vi "Monitored Actor Switcher.vi"() -> ()   [LabVIEW 2017]
doc: "Provides an easy way to switch actors between monitored actors and reular actors\n\nCopyright: Hill\nAuthored by: Derek Trepanier"
panel:
  in  "Non Actors":i32[](listbox)
  in  "All Actors to Non":bool
  in  "Actor to Non":bool
  in  "All Non to Actors":bool
  in  "Non to Actor":bool
  in  "Actors":i32[](listbox) caption="MGI-Monitored Actor Core.lvlib:Actor Monitor.lvclass"
  in  "All Mon to Actors":bool
  in  "Mon to Actor":bool
  in  "All Actors to Mon":bool
  in  "Actor To Mon":bool
  in  "Monitored Actors":i32[](listbox) caption="Example Actor.lvlib:Example Actor.lvclass"
  in  "Include Items in Dependancies?":bool
  in  "Cancel":bool
  in  "Save":bool
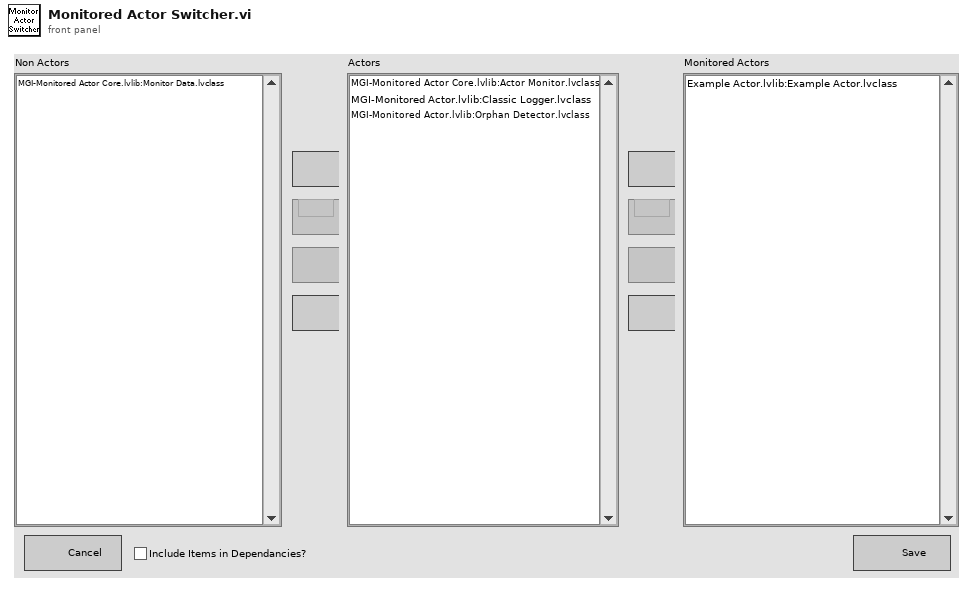
[diagram p1: front panel]
types:
  T1 = enum8{"Enabled", "Disabled", "Disabled and Grayed Out"}
  T2 = typedef "LVPoint32TypeDef.ctl" = cluster{"Horizontal":i32, "Vertical":i32}
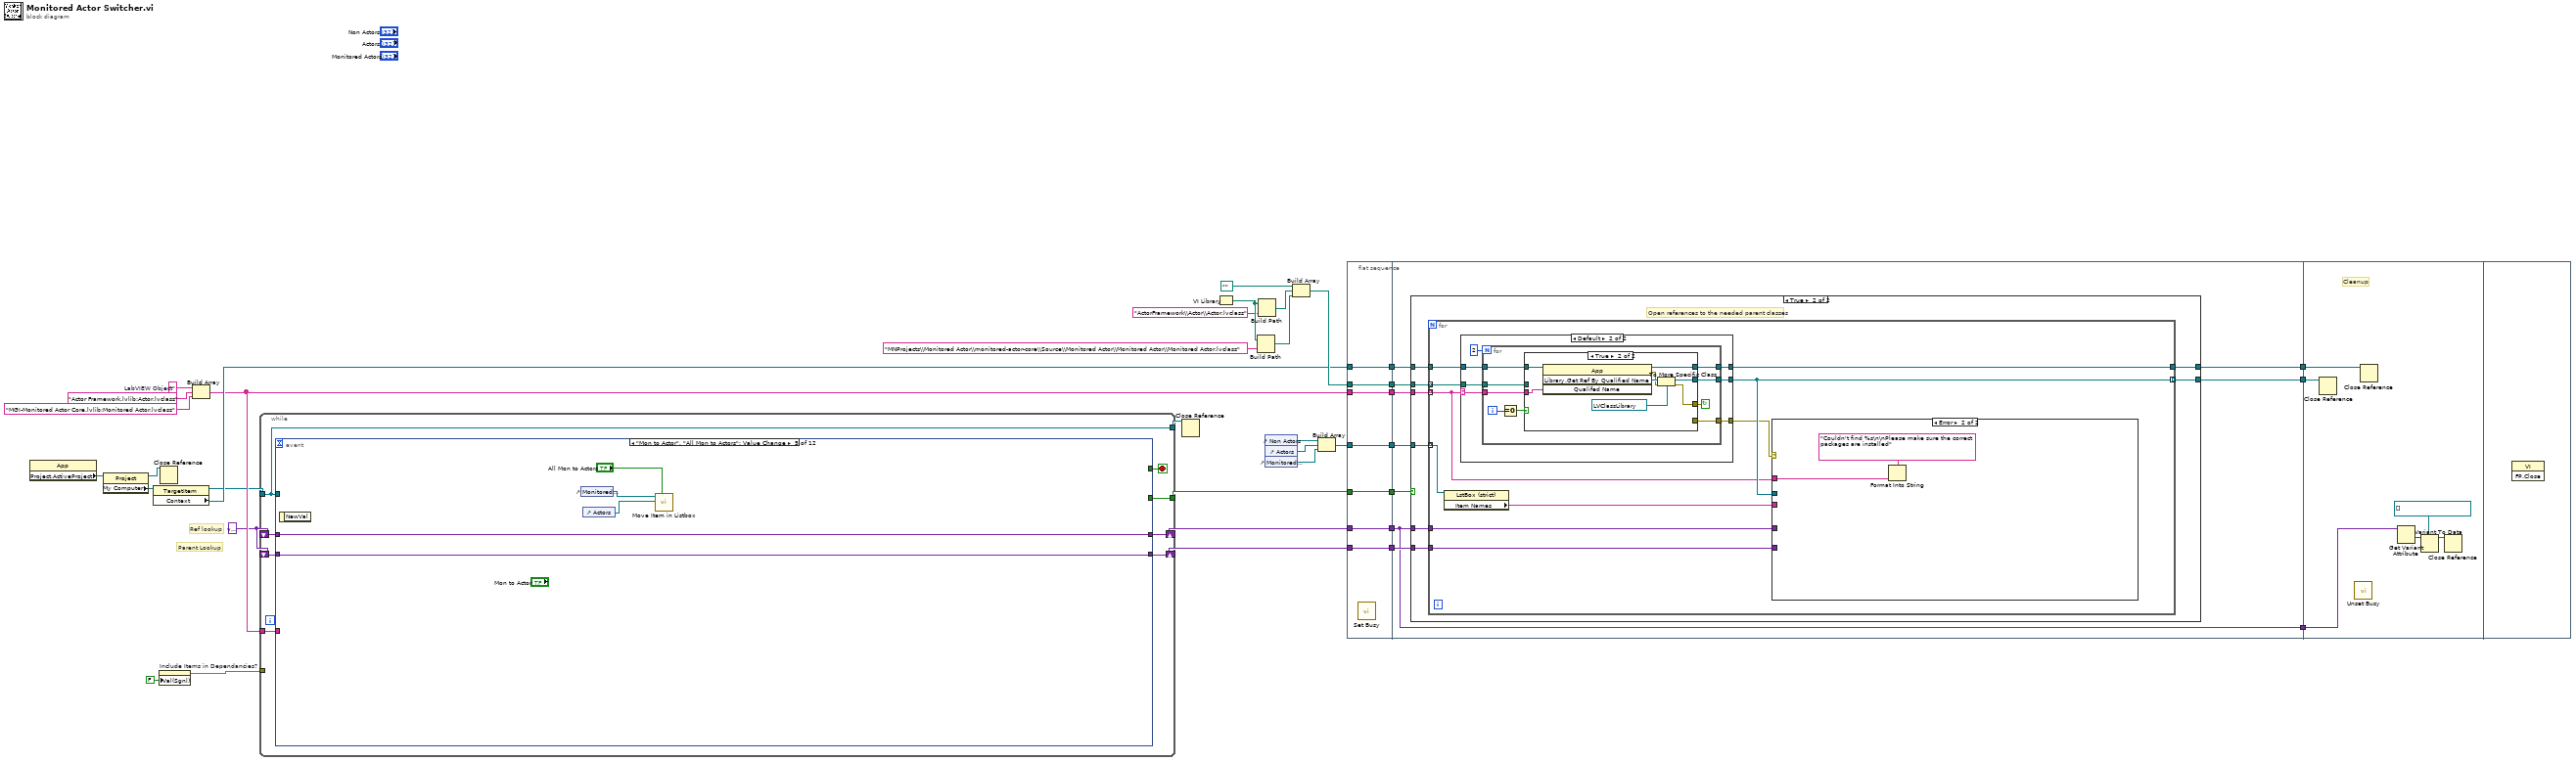
[diagram p0: block diagram]
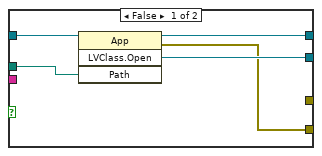
[diagram p4: hidden frame]
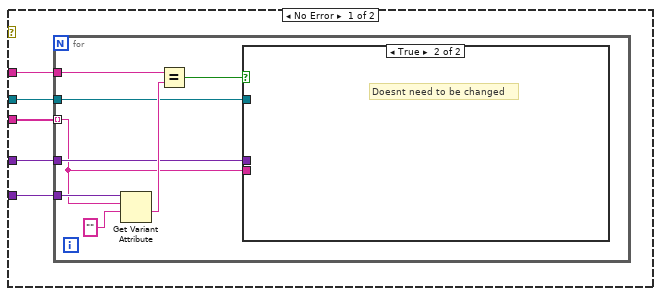
[diagram p5: hidden frame]
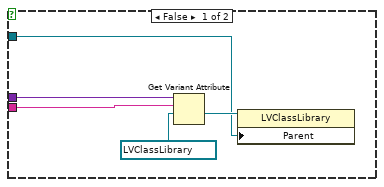
[diagram p6: hidden frame]
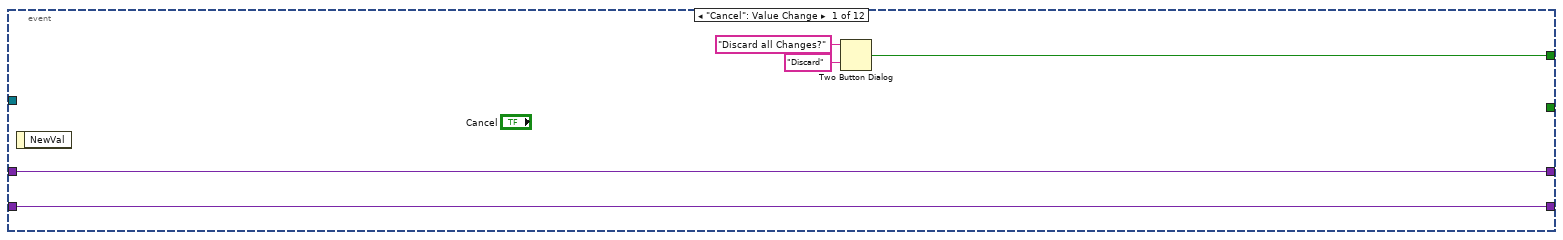
[diagram p7: hidden frame]
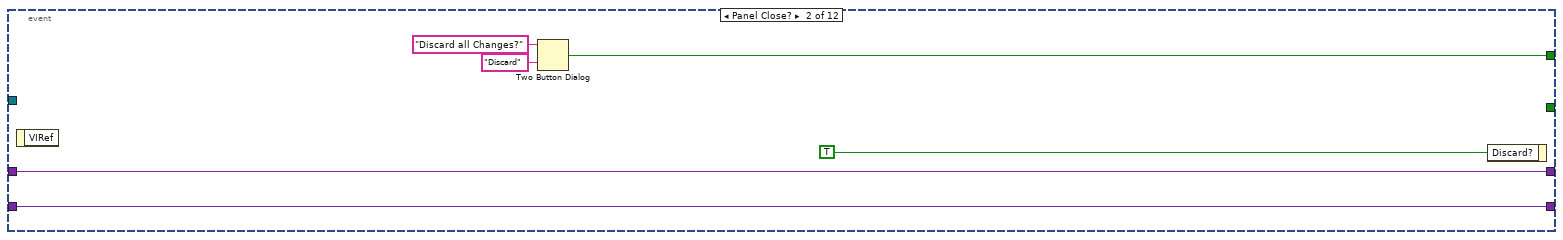
[diagram p8: hidden frame]
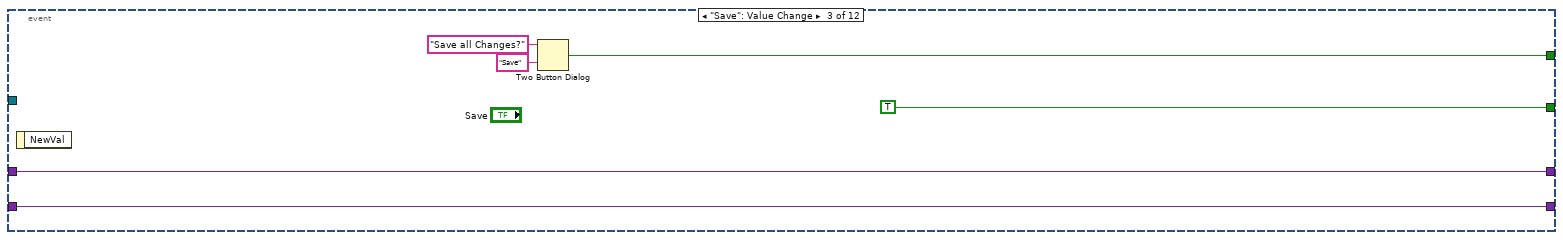
[diagram p9: hidden frame]
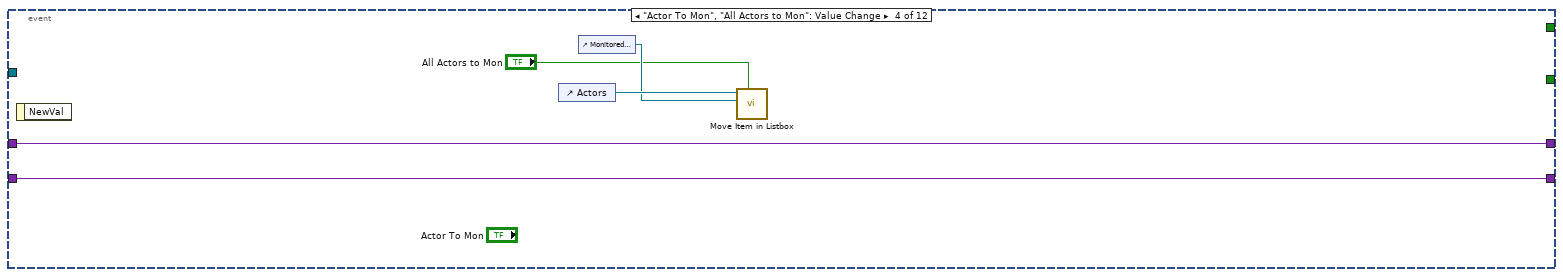
[diagram p10: hidden frame]
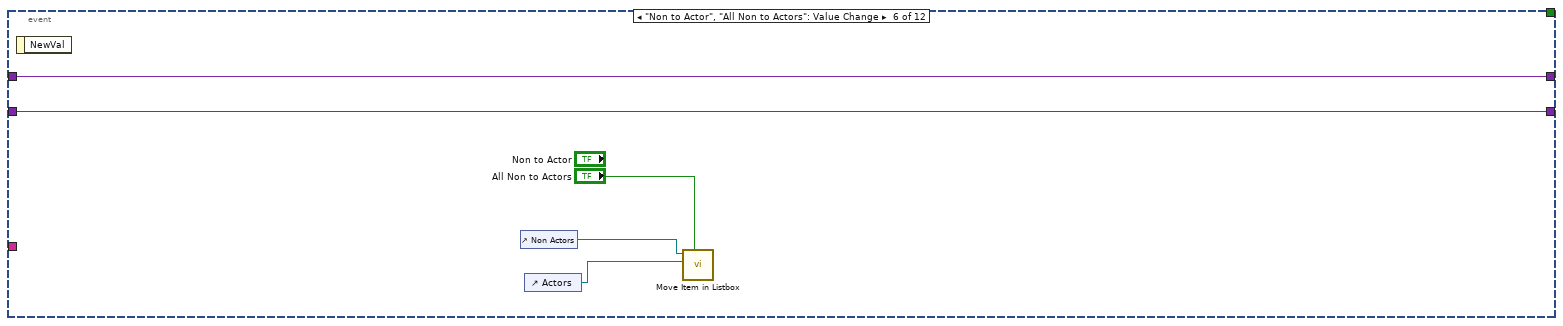
[diagram p11: hidden frame]
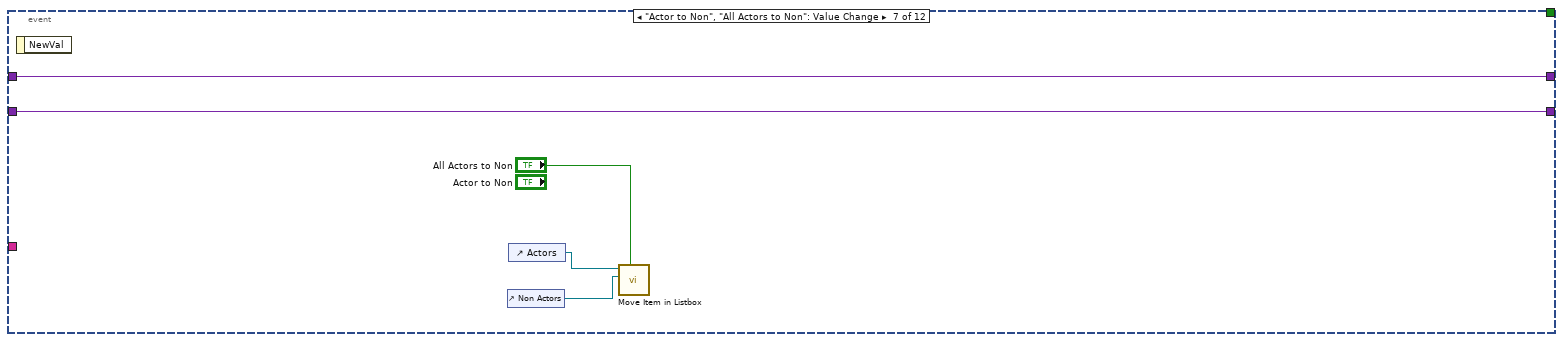
[diagram p12: hidden frame]
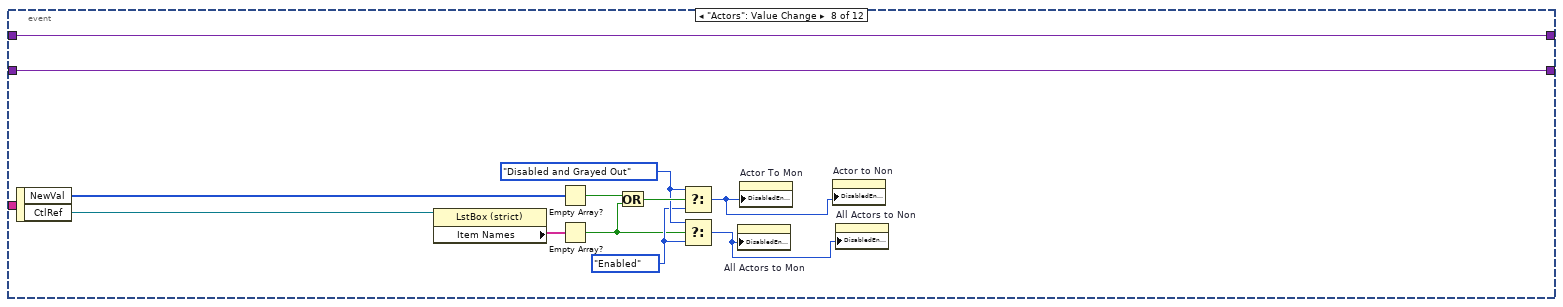
[diagram p13: hidden frame]
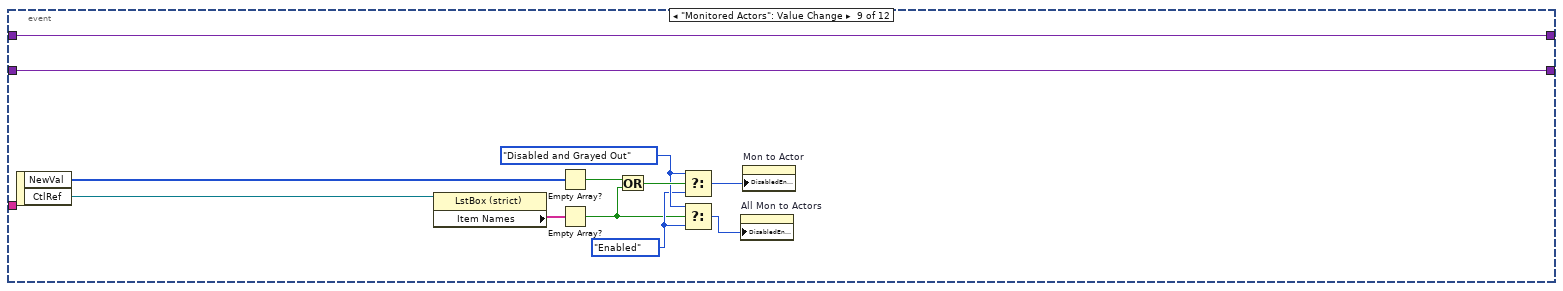
[diagram p14: hidden frame]
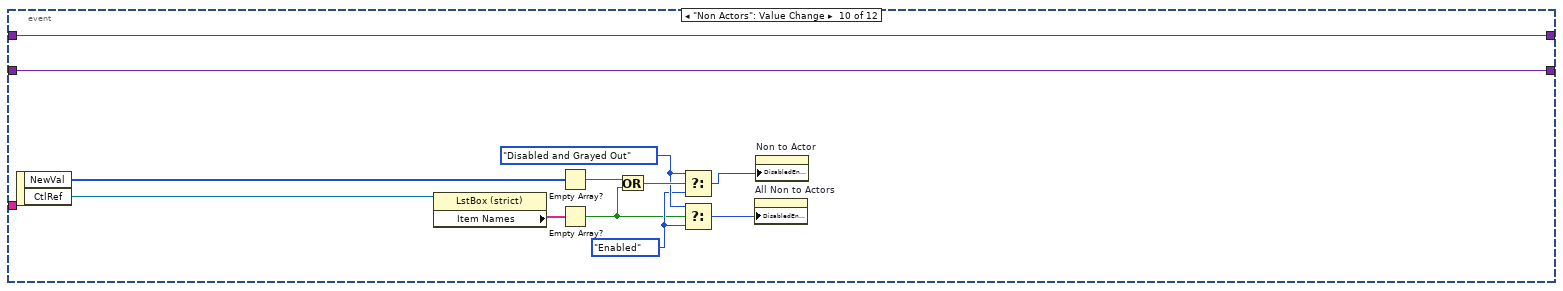
[diagram p15: hidden frame]
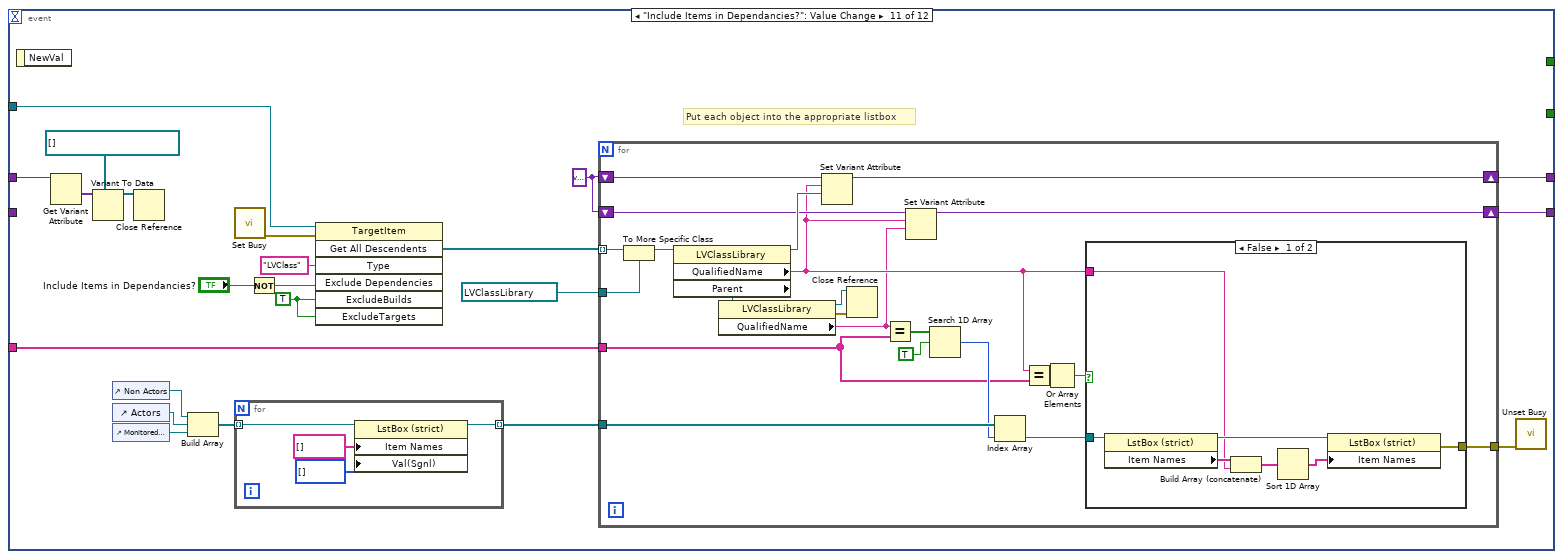
[diagram p16: hidden frame]
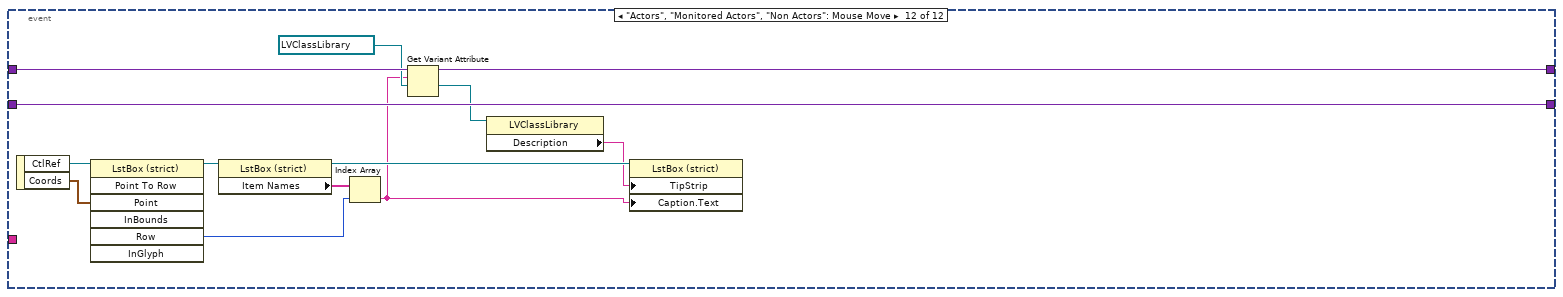
[diagram p18: hidden frame]
diagram:
  w1 = variant ("Variant")
  w11 = ""  # LabVIEW Object
  # "Parent Lookup"
  # "Ref lookup"
  n1 = property class="App"() -> ("Project.ActiveProject"=w37:refnum<vi>)  [unwired: 2 in, 2 out]
  n2 = property class="Project"(reference=w37) -> (reference out=w35:refnum<vi>, "My Computer"=w36:refnum<vi>)  [unwired: 1 in, 1 out]
  n3 = property class="TargetItem"(reference=w36) -> (reference out=w5:refnum<vi>, "Context"=w30:refnum<vi>)  [unwired: 1 in, 1 out]
  n4 = property on="Include Items in Dependancies?" class="Bool (strict)"("Val(Sgnl)"=FALSE ("Value (Signaling)")) -> (error out=w3:errorcluster)  [unwired: 2 in, 1 out]
  n5 = Close Reference(reference=w35) -> ()  [unwired: 1 in, 1 out]
  n6 = Build Array(w11, "Actor Framework.lvlib:Actor.lvclass" ("Qualified Name"), "MGI-Monitored Actor Core.lvlib:Monitored Actor.lvclass" ("Qualified Name")) -> (w8:string[])
  n7 = while {
    tunnel: [w44] -> w22
    tunnel: w8 -> [w43]
    tunnel: w5 -> [w40]
    tunnel: w3 -> [_]
    tunnel: [w40] -> w2
    shift-right: [w42] -> w7
    shift-left: w1 -> [w38]
    shift-right: [w41] -> w6
    shift-left: w1 -> [w39]
    stop <- w45 stop-if-true
    n8 = event shown="[4] \"Mon to Actor\", \"All Mon to Actors\": Value Change" {
      selector: _ -> [_ _ _ _ _ _ _ _ _ _ _ _]
      dyn-events: _ -> [_ _ _ _ _ _ _ _ _ _ _ _]
      timeout: _ -> [_ _ _ _ _ _ _ _ _ _ _ _]
      tunnel: [w50 w56 w62 _ _ _ _ _ _ _ _ _] -> w45
      tunnel: [_ _ TRUE _ _ _ _ _ _ _ _ _] -> w44
      tunnel: w43 -> [_ _ _ _ _ _ _ _ _ _ w130 _]
      tunnel: [w47 w52 w58 w64 w69 w74 w79 w84 w96 w108 w128 w179] -> w42
      tunnel: [w46 w51 w57 w63 w68 w73 w78 w83 w95 w107 w127 w186] -> w41
      tunnel: w40 -> [_ _ _ _ _ _ _ _ _ _ w125 _]
      tunnel: w39 -> [w46 w51 w57 w63 w68 w73 w78 w83 w95 w107 _ w186]
      tunnel: w38 -> [w47 w52 w58 w64 w69 w74 w79 w84 w96 w108 w119 w180]
      event "Cancel": Value Change {
        n9 = event-data() -> ()  [unwired: 1 in, 1 out]
        n10 = Two Button Dialog(message="Discard all Changes?", 2:"Discard" ("T button name (\"OK\")")) -> (T button?=w50:bool)  [unwired: 1 in]
      }
      event Panel Close? {
        n11 = event-data() -> ()  [unwired: 1 in, 1 out]
        n12 = Two Button Dialog(message="Discard all Changes?", 2:"Discard" ("T button name (\"OK\")")) -> (T button?=w56:bool)  [unwired: 1 in]
        n13 = event-data("Discard?"=TRUE) -> ()  [unwired: 1 in, 1 out]
      }
      event "Save": Value Change {
        n14 = event-data() -> ()  [unwired: 1 in, 1 out]
        n15 = Two Button Dialog(message="Save all Changes?", 2:"Save" ("T button name (\"OK\")")) -> (T button?=w62:bool)  [unwired: 1 in]
      }
      event "Actor To Mon", "All Actors to Mon": Value Change {
        n16 = event-data() -> ()  [unwired: 1 in, 1 out]
        n17 = control-ref of="Actors"() -> (w67:refnum<vi>)
        n18 = control-ref of="Monitored Actors"() -> (w66:refnum<vi>)
        n19 = call "Move Item in Listbox.vi"("Move All Items? (f)"="All Actors to Mon", "Destination Lisbox"=w66, "Source Listbox"=w67) -> ()  [unwired: 9 in]
      }
      event "Mon to Actor", "All Mon to Actors": Value Change {
        n20 = event-data() -> ()  [unwired: 1 in, 1 out]
        n21 = control-ref of="Monitored Actors"() -> (w70:refnum<vi>)
        n22 = control-ref of="Actors"() -> (w71:refnum<vi>)
        n23 = call "Move Item in Listbox.vi"("Move All Items? (f)"="All Mon to Actors", "Destination Lisbox"=w71, "Source Listbox"=w70) -> ()  [unwired: 9 in]
      }
      event "Non to Actor", "All Non to Actors": Value Change {
        n24 = event-data() -> ()  [unwired: 1 in, 1 out]
        n25 = control-ref of="Non Actors"() -> (w77:refnum<vi>)
        n26 = control-ref of="Actors"() -> (w76:refnum<vi>)
        n27 = call "Move Item in Listbox.vi"("Move All Items? (f)"="All Non to Actors", "Destination Lisbox"=w76, "Source Listbox"=w77) -> ()  [unwired: 9 in]
      }
      event "Actor to Non", "All Actors to Non": Value Change {
        n28 = event-data() -> ()  [unwired: 1 in, 1 out]
        n29 = control-ref of="Non Actors"() -> (w80:refnum<vi>)
        n30 = control-ref of="Actors"() -> (w81:refnum<vi>)
        n31 = call "Move Item in Listbox.vi"("Move All Items? (f)"="All Actors to Non", "Destination Lisbox"=w80, "Source Listbox"=w81) -> ()  [unwired: 9 in]
      }
      event "Actors": Value Change {
        w88 = T1."Enabled" ("Disabled")
        w89 = T1."Disabled and Grayed Out" ("Disabled")
        n32 = event-data() -> ("NewVal"=w94:i32[], "CtlRef"=w93:refnum<vi>)  [unwired: 1 in]
        n33 = property class="LstBox (strict)"(reference=w93) -> ("Item Names"=w92:string[])  [unwired: 1 in, 2 out]
        n34 = Empty Array?(array=w94) -> (empty?=w91:bool)
        n35 = Empty Array?(array=w92) -> (empty?=w87:bool)
        n36 = Or(x=w91, y=w87) -> (x .or. y?=w90:bool)
        n37 = Select(t=w89, s=w90, f=w88) -> (s? t:f=w85:T1)
        n38 = Select(t=w89, s=w87, f=w88) -> (s? t:f=w86:T1)
        n39 = property on="All Actors to Mon" class="Bool"("DisabledEnum"=w86) -> ()  [unwired: 2 in, 2 out]
        n40 = property on="Actor To Mon" class="Bool"("DisabledEnum"=w85) -> ()  [unwired: 2 in, 2 out]
        n41 = property on="Actor to Non" class="Bool"("DisabledEnum"=w85) -> ()  [unwired: 2 in, 2 out]
        n42 = property on="All Actors to Non" class="Bool"("DisabledEnum"=w86) -> ()  [unwired: 2 in, 2 out]
      }
      event "Monitored Actors": Value Change {
        w100 = T1."Enabled" ("Disabled")
        w101 = T1."Disabled and Grayed Out" ("Disabled")
        n43 = event-data() -> ("NewVal"=w106:i32[], "CtlRef"=w105:refnum<vi>)  [unwired: 1 in]
        n44 = property class="LstBox (strict)"(reference=w105) -> ("Item Names"=w104:string[])  [unwired: 1 in, 2 out]
        n45 = Empty Array?(array=w106) -> (empty?=w103:bool)
        n46 = Empty Array?(array=w104) -> (empty?=w99:bool)
        n47 = Or(x=w103, y=w99) -> (x .or. y?=w102:bool)
        n48 = Select(t=w101, s=w102, f=w100) -> (s? t:f=w98:T1)
        n49 = Select(t=w101, s=w99, f=w100) -> (s? t:f=w97:T1)
        n50 = property on="All Mon to Actors" class="Bool"("DisabledEnum"=w97) -> ()  [unwired: 2 in, 2 out]
        n51 = property on="Mon to Actor" class="Bool"("DisabledEnum"=w98) -> ()  [unwired: 2 in, 2 out]
      }
      event "Non Actors": Value Change {
        w112 = T1."Enabled" ("Disabled")
        w113 = T1."Disabled and Grayed Out" ("Disabled")
        n52 = event-data() -> ("NewVal"=w118:i32[], "CtlRef"=w117:refnum<vi>)  [unwired: 1 in]
        n53 = property class="LstBox (strict)"(reference=w117) -> ("Item Names"=w116:string[])  [unwired: 1 in, 2 out]
        n54 = Empty Array?(array=w118) -> (empty?=w115:bool)
        n55 = Empty Array?(array=w116) -> (empty?=w111:bool)
        n56 = Or(x=w115, y=w111) -> (x .or. y?=w114:bool)
        n57 = Select(t=w113, s=w114, f=w112) -> (s? t:f=w109:T1)
        n58 = Select(t=w113, s=w111, f=w112) -> (s? t:f=w110:T1)
        n59 = property on="All Non to Actors" class="Bool"("DisabledEnum"=w110) -> ()  [unwired: 2 in, 2 out]
        n60 = property on="Non to Actor" class="Bool"("DisabledEnum"=w109) -> ()  [unwired: 2 in, 2 out]
      }
      event "Include Items in Dependancies?": Value Change {
        w140 = variant ("Variant")
        w139 = TRUE ("ExcludeDependencies")
        # "Put each object into the appropriate listbox"
        n61 = event-data() -> ()  [unwired: 1 in, 1 out]
        n62 = Get Variant Attribute(Variant=w119) -> (values=w121:variant[])  [unwired: 3 in, 3 out]
        n63 = Variant To Data(type=refnum<vi>[] [] ("Children In Memory[]"), Variant=w121) -> (data=w120:refnum<vi>[])  [unwired: 1 in, 1 out]
        n64 = control-ref of="Non Actors"() -> (w133:refnum<vi>)
        n65 = control-ref of="Actors"() -> (w131:refnum<vi>)
        n66 = control-ref of="Monitored Actors"() -> (w132:refnum<vi>)
        n67 = Close Reference(reference=w120) -> ()  [unwired: 1 in, 1 out]
        n68 = Build Array(w133, w131, w132) -> (w137:refnum<vi>[])
        n69 = call <vilib>:"Set Busy.vi"() -> ("error out"=w126:errorcluster)  [unwired: 10 in, 1 out]
        n70 = for {
          tunnel: w137 -> [w144] mode=indexing
          tunnel: [w143] -> w138 mode=indexing
          n71 = property class="LstBox (strict)"(reference=w144, "Item Names"=string[] [], "Val(Sgnl)"=i32[] [] ("Value (Signaling)")) -> (reference out=w143:refnum<vi>)  [unwired: 1 in, 1 out]
        }
        n72 = Not(x="Include Items in Dependancies?") -> (.not. x?=w123:bool)
        n73 = invoke class="TargetItem" method="Get All Descendents"(reference=w125, error in=w126, "Type"="LVClass", "Exclude Dependencies"=w123, "ExcludeBuilds"=w139, "ExcludeTargets"=w139) -> ("All Descendents"=w129:refnum<vi>[])  [unwired: 1 in, 6 out]
        n74 = for {
          tunnel: w138 -> [w166]
          tunnel: w129 -> [w163] mode=indexing
          tunnel: refnum<vi> refnum ("Library:Get Ref By Qualified Name") -> [w161]
          tunnel: [w158] -> w136
          tunnel: w130 -> [w154]
          shift-right: [w145] -> w128
          shift-left: w140 -> [w151]
          shift-right: [w146] -> w127
          shift-left: w140 -> [w149]
          n75 = To More Specific Class(target class=w161, reference=w163) -> (specific class reference=w162:refnum<vi>)  [unwired: 1 in, 1 out]
          n76 = property class="LVClassLibrary"(reference=w162) -> (reference out=w150:refnum<vi>, "QualifiedName"=w148:string, "Parent"=w157:refnum<vi>)  [unwired: 1 in, 1 out]
          n77 = property class="LVClassLibrary"(reference=w157) -> (reference out=w155:refnum<vi>, error out=w156:errorcluster, "QualifiedName"=w147:string)  [unwired: 1 in]
          n78 = Set Variant Attribute(Variant=w151, name=w148, value=w150) -> (Variant out=w145:variant)  [unwired: 1 in, 2 out]
          n79 = Close Reference(reference=w155, error in (no error)=w156) -> ()  [unwired: 1 out]
          n80 = Equal?(x=w147, y=w154) -> (x = y?=w165:bool[])
          n81 = Set Variant Attribute(Variant=w149, name=w148, value=w147) -> (Variant out=w146:variant)  [unwired: 1 in, 2 out]
          n82 = Search 1D Array(1D array=w165, element=TRUE) -> (index of element=w160:i32)  [unwired: 1 in]
          n83 = Index Array(array=w166, index=w160) -> (element=w159:refnum<vi>)
          n84 = Equal?(x=w148, y=w154) -> (x = y?=w153:bool[])
          n85 = Or Array Elements(Boolean array=w153) -> (logical OR=w152:bool)
          n86 = case shown="False" w152 {
            tunnel: w159 -> [w173 _]
            tunnel: w148 -> [w170 _]
            tunnel: [w167 _] -> w158
            frame False {
              n87 = property class="LstBox (strict)"(reference=w173) -> (reference out=w172:refnum<vi>, "Item Names"=w171:string[])  [unwired: 1 in, 1 out]
              n88 = Build Array (concatenate)(w171, w170) -> (w169:string[])
              n89 = Sort 1D Array(array=w169) -> (sorted array=w168:string[])
              n90 = property class="LstBox (strict)"(reference=w172, "Item Names"=w168) -> (error out=w167:errorcluster)  [unwired: 1 in, 1 out]
            }
            frame True {
            }
          }
        }
        n91 = call <vilib>:"Unset Busy.vi"("error in (no error)"=w136) -> ()  [unwired: 10 in, 1 out]
      }
      event "Actors", "Monitored Actors", "Non Actors": Mouse Move {
        n92 = event-data() -> ("CtlRef"=w185:refnum<vi>, "Coords"=w183:T2)  [unwired: 1 in]
        n93 = invoke class="LstBox (strict)" method="Point To Row"(reference=w185, "Point"=w183) -> (reference out=w184:refnum<vi>, "Row"=w181:i32)  [unwired: 5 in, 5 out]
        n94 = property class="LstBox (strict)"(reference=w184) -> (reference out=w176:refnum<vi>, "Item Names"=w182:string[])  [unwired: 1 in, 1 out]
        n95 = Index Array(array=w182, index=w181) -> (element=w174:string)
        n96 = Get Variant Attribute(Variant=w180, name=w174, default value (empty Variant)=refnum<vi> refnum ("Library:Get Ref By Qualified Name")) -> (duplicate Variant=w179:variant, value=w177:refnum<vi>)  [unwired: 1 in, 2 out]
        n97 = property class="LVClassLibrary"(reference=w177) -> ("Description"=w175:string)  [unwired: 1 in, 2 out]
        n98 = property class="LstBox (strict)"(reference=w176, "TipStrip"=w175, "Caption.Text"=w174) -> ()  [unwired: 1 in, 2 out]
      }
    }
  }
  n99 = Close Reference(reference=w2) -> ()  [unwired: 1 in, 1 out]
  n100 = VI Library() -> (path=w32:path)
  n101 = Build Path(base path=w32, name or relative path="MNProjects\\Monitored Actor\\monitored-actor-core\\Source\\Monitored Actor\\Monitored Actor\\Monitored Actor.lvclass") -> (appended path=w9:path)
  n102 = Build Path(base path=w32, name or relative path="ActorFramework\\Actor\\Actor.lvclass") -> (appended path=w33:path)
  n103 = control-ref of="Non Actors"() -> (w28:refnum<vi>)
  n104 = control-ref of="Actors"() -> (w27:refnum<vi>)
  n105 = control-ref of="Monitored Actors"() -> (w26:refnum<vi>)
  n106 = Build Array(path "" ("path"), w33, w9) -> (w31:path[])
  n107 = Build Array(w28, w27, w26) -> (w25:refnum<vi>[])
  n108 = flat-sequence {
    tunnel: w22 -> [w187]
    tunnel: w25 -> [w188]
    tunnel: w8 -> [w189]
    tunnel: w6 -> [w190]
    tunnel: w30 -> [w191]
    tunnel: w31 -> [w192]
    tunnel: w7 -> [w193]
    tunnel: [w193] -> w21
    tunnel: [w192] -> w20
    tunnel: [w191] -> w19
    tunnel: [w190] -> w18
    tunnel: [w189] -> w17
    tunnel: [w188] -> w16
    tunnel: [w187] -> w15
    tunnel: [w199] -> w29
    tunnel: [w196] -> w24
    tunnel: [w195] -> w23
    tunnel: w21 -> [w195]
    tunnel: w20 -> [w202]
    tunnel: w19 -> [w201]
    tunnel: w18 -> [w198]
    tunnel: w17 -> [w200]
    tunnel: w16 -> [w197]
    tunnel: w15 -> [w194]
    tunnel: w29 -> [w273]
    tunnel: w24 -> [w272]
    tunnel: w23 -> [w274]
    frame #0 {
      n109 = call <vilib>:"Set Busy.vi"() -> ()  [unwired: 10 in, 2 out]
    }
    frame #1 {
      n110 = case shown="True" w194 {
        tunnel: w202 -> [_ w211]
        tunnel: w201 -> [w203 w210]
        tunnel: w200 -> [_ w209]
        tunnel: [w203 w208] -> w199
        tunnel: w198 -> [_ w207]
        tunnel: w197 -> [_ w206]
        tunnel: [_ w205] -> w196
        tunnel: w195 -> [_ w204]
        frame False {
          # "Discard clicked, don't change anything"
        }
        frame True {
          # "Open references to the needed parent classes"
          n111 = for {
            tunnel: w211 -> [w220] mode=indexing
            tunnel: w210 -> [w221]
            tunnel: [w219] -> w208
            tunnel: w209 -> [w214] mode=indexing
            tunnel: w207 -> [w218]
            tunnel: w204 -> [w216]
            tunnel: w206 -> [w217] mode=indexing
            tunnel: [w215] -> w205 mode=indexing
            n112 = property class="LstBox (strict)"(reference=w217) -> ("Item Names"=w212:string[])  [unwired: 1 in, 2 out]
            n113 = case shown="Default" w214 {
              selector: w214 -> [_ w224]
              tunnel: w221 -> [w222 w229]
              tunnel: w220 -> [_ w228]
              tunnel: [w222 w227] -> w219
              tunnel: [_ w225] -> w215
              tunnel: [_ w223] -> w213
              frame "" {
                # "This is the base LVObj"
              }
              frame Default {
                n114 = for {
                  N: 2 -> [_]
                  tunnel: w229 -> [w238]
                  tunnel: w228 -> [w237]
                  tunnel: [w236] -> w225
                  tunnel: [w235] -> w227
                  tunnel: w224 -> [w232]
                  tunnel: [w230] -> w223
                  i -> [w233]
                  stop <- w231 continue-if-true
                  n115 = Equal To 0?(x=w233) -> (x = 0?=w234:bool)
                  n116 = case shown="True" w234 {
                    tunnel: w238 -> [w243 w251]
                    tunnel: w237 -> [w242 _]
                    tunnel: [w241 w247] -> w236
                    tunnel: [w240 w250] -> w235
                    tunnel: w232 -> [_ w248]
                    tunnel: [_ w244] -> w231
                    tunnel: [w239 _] -> w230
                    frame False {
                      n117 = invoke class="App" method="LVClass.Open"(reference=w243, "Path"=w242) -> (reference out=w240:refnum<vi>, error out=w239:errorcluster, "LVClass.Open"=w241:refnum<vi>)  [unwired: 2 in, 1 out]
                    }
                    frame True {
                      n118 = invoke class="App" method="Library.Get Ref By Qualified Name"(reference=w251, "Qualifed Name"=w248) -> (reference out=w250:refnum<vi>, error out=w245:errorcluster, "Library.Get Ref By Qualified Name"=w249:refnum<vi>)  [unwired: 2 in, 1 out]
                      n119 = To More Specific Class(target class=refnum<vi> refnum ("Library:Get Ref By Qualified Name"), reference=w249, error in=w245) -> (specific class reference=w247:refnum<vi>, error out=w244:errorcluster)
                    }
                  }
                }
              }
            }
            n120 = case shown="Error" w213 {
              tunnel: w218 -> [w256 _]
              tunnel: w212 -> [w255 _]
              tunnel: w216 -> [w254 _]
              tunnel: w215 -> [w253 _]
              tunnel: w214 -> [w252 w270]
              frame No Error {
                n121 = for {
                  tunnel: w256 -> [w264]
                  tunnel: w255 -> [w258] mode=indexing
                  tunnel: w254 -> [w259]
                  tunnel: w252 -> [w262]
                  tunnel: w253 -> [w257]
                  n122 = Get Variant Attribute(Variant=w264, name=w258, default value (empty Variant)="") -> (value=w261:string)  [unwired: 1 in, 3 out]
                  n123 = Equal?(x=w262, y=w261) -> (x = y?=w260:bool)
                  n124 = case shown="True" w260 {
                    tunnel: w259 -> [w269 _]
                    tunnel: w258 -> [w267 _]
                    tunnel: w257 -> [w265 _]
                    frame False {
                      n125 = Get Variant Attribute(Variant=w269, name=w267, default value (empty Variant)=refnum<vi> refnum ("Library:Get Ref By Qualified Name")) -> (value=w266:refnum<vi>)  [unwired: 1 in, 3 out]
                      n126 = property class="LVClassLibrary"(reference=w266, "Parent"=w265) -> ()  [unwired: 1 in, 2 out]
                    }
                    frame True {
                      # "Doesnt need to be changed"
                    }
                  }
                }
              }
              frame Error {
                n127 = Format Into String(format string="Couldn't find %s\n\nPlease make sure the correct packages are installed", w270) -> ()  [unwired: 2 in, 2 out]
              }
            }
          }
        }
      }
    }
    frame #2 {
      # "Cleanup"
      n128 = Close Reference(reference=w272) -> ()  [unwired: 1 in, 1 out]
      n129 = call <vilib>:"Unset Busy.vi"() -> ()  [unwired: 11 in, 1 out]
      n130 = Close Reference(reference=w273) -> ()  [unwired: 1 in, 1 out]
      n131 = Get Variant Attribute(Variant=w274) -> (values=w276:variant[])  [unwired: 3 in, 3 out]
      n132 = Variant To Data(type=refnum<vi>[] [] ("Children In Memory[]"), Variant=w276) -> (data=w275:refnum<vi>[])  [unwired: 1 in, 1 out]
      n133 = Close Reference(reference=w275) -> ()  [unwired: 1 in, 1 out]
    }
    frame #3 {
      n134 = invoke class="VI" method="FP.Close"() -> ()  [unwired: 3 in, 3 out]
    }
  }
